vi "spot_shape.vi"(1 "Spot":T1 {"Amplitude Correction" step=0.1; "Line Trapping"."Phase Gradient" step=0.05; "Line Trapping"."Vector"."x" step=1e-06 format="%#_6p"; "Line Trapping"."Vector"."y" step=1e-06 format="%#_6p"; "Line Trapping"."Vector"."z" step=1e-06 format="%#_6p"; "NA Position"."r" step=1e-06; "NA Position"."y" step=1e-06; "NA Position"."x" step=1e-06; "Position"."z" step=1e-06; "Position"."y" step=1e-06; "Position"."x" step=1e-06; "Phase" step=0.7753; "Intensity" step=0.1}) -> (0 "Spot Shape":enum32{"Normal", "Line", "NA", "Mixed"}(ring))   [LabVIEW 2010]
uses:
  spot.ctl
  line_trapping.ctl
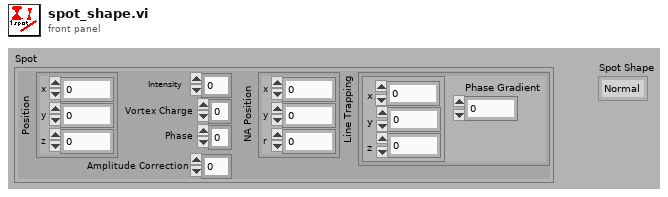
[diagram p1: front panel]
types:
  T1 = typedef "spot.ctl" = cluster{"Position":cluster{"x":dbl, "y":dbl, "z":dbl}, "Intensity":dbl, "Vortex Charge":i8, "Phase":dbl, "NA Position":cluster{"x":dbl, "y":dbl, "r":dbl}, "Line Trapping":T2, "Amplitude Correction":dbl}
  T2 = typedef "line_trapping.ctl" = cluster{"Vector":cluster{"x":dbl, "y":dbl, "z":dbl}, "Phase Gradient":dbl}
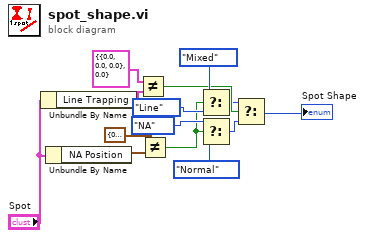
[diagram p0: block diagram]
diagram:
  n1 = Unbundle By Name("Spot") -> ("Line Trapping"=w1:T2)
  n2 = Unbundle By Name("Spot") -> ("NA Position"=w4:cluster{"x":dbl, "y":dbl, "r":dbl})
  n3 = Not Equal?(x=T2 {"Vector"={"x"=0.0, "y"=0.0, "z"=0.0}, "Phase Gradient"=0.0} ("Line Trapping"), y=w1) -> (x != y?=w8:bool)
  n4 = Not Equal?(x=cluster{"x":dbl, "y":dbl, "r":dbl} {"x"=0.0, "y"=0.0, "r"=1.0}, y=w4) -> (x != y?=w9:bool)
  n5 = Select(t=enum32{"Normal", "Line", "NA", "Mixed"}."Mixed" ("f"), s=w9, f=enum32{"Normal", "Line", "NA", "Mixed"}."Line" ("Spot Shape")) -> (s? t:f=w6:enum32{"Normal", "Line", "NA", "Mixed"})
  n6 = Select(t=enum32{"Normal", "Line", "NA", "Mixed"}."NA" ("Spot Shape"), s=w9, f=enum32{"Normal", "Line", "NA", "Mixed"}."Normal") -> (s? t:f=w7:enum32{"Normal", "Line", "NA", "Mixed"})
  n7 = Select(t=w6, s=w8, f=w7) -> (s? t:f=→"Spot Shape":enum32{"Normal", "Line", "NA", "Mixed"})
